vi "Draw Angle Line.vi"(9 "BG Image Property In":T1={"Radius"=[], "Plot Area Bounds"={"Left"=0, "Top"=0, "Right"=0, "Bottom"=0}, "Center position"={"X"=0, "Y"=0}, "Flip?"=FALSE, "Major Gird Color"=10066176, "Minor Gird Color"=5000192}, 11 "Picture In":picture) -> (1 "BG Image Property Out":T1={"Radius"=[], "Plot Area Bounds"={"Left"=0, "Top"=0, "Right"=0, "Bottom"=0}, "Center position"={"X"=0, "Y"=0}, "Flip?"=FALSE, "Major Gird Color"=10066176, "Minor Gird Color"=5000192}, 3 "Picture Out":picture)   [LabVIEW 2020, in "2D Compass.lvclass"]
uses:
  <vilib>/Math Plots/2D Math Plots/2D Compass/2D Compass/2D Compass.lvclass
  <vilib>/Math Plots/2D Math Plots/2D Compass/2D Compass/Typedef/BG Image Property.ctl
  <vilib>/Utility/miscctls.llb/LVRectTypeDef.ctl
panel:
  in  "Default Angle Array":cluster{"Angle":dbl, "Min Radius":i16}[](array[cluster])=[{"Angle"=0.0, "Min Radius"=0}, {"Angle"=15.0, "Min Radius"=25}, {"Angle"=30.0, "Min Radius"=25}, {"Angle"=45.0, "Min Radius"=10}, {"Angle"=60.0, "Min Radius"=25}, {"Angle"=75.0, "Min Radius"=25}]
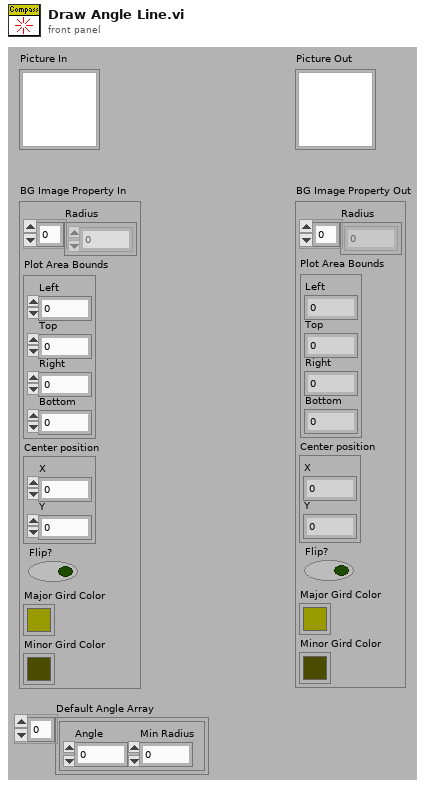
[diagram p1: front panel]
types:
  T1 = typedef "2D Compass.lvclass/BG Image Property.ctl" = cluster{"Radius":i16[], "Plot Area Bounds":T2, "Center position":cluster{"X":i16, "Y":i16}, "Flip?":bool, "Major Gird Color":u32, "Minor Gird Color":u32}
  T2 = typedef "LVRectTypeDef.ctl" = cluster{"Left":i16, "Top":i16, "Right":i16, "Bottom":i16}
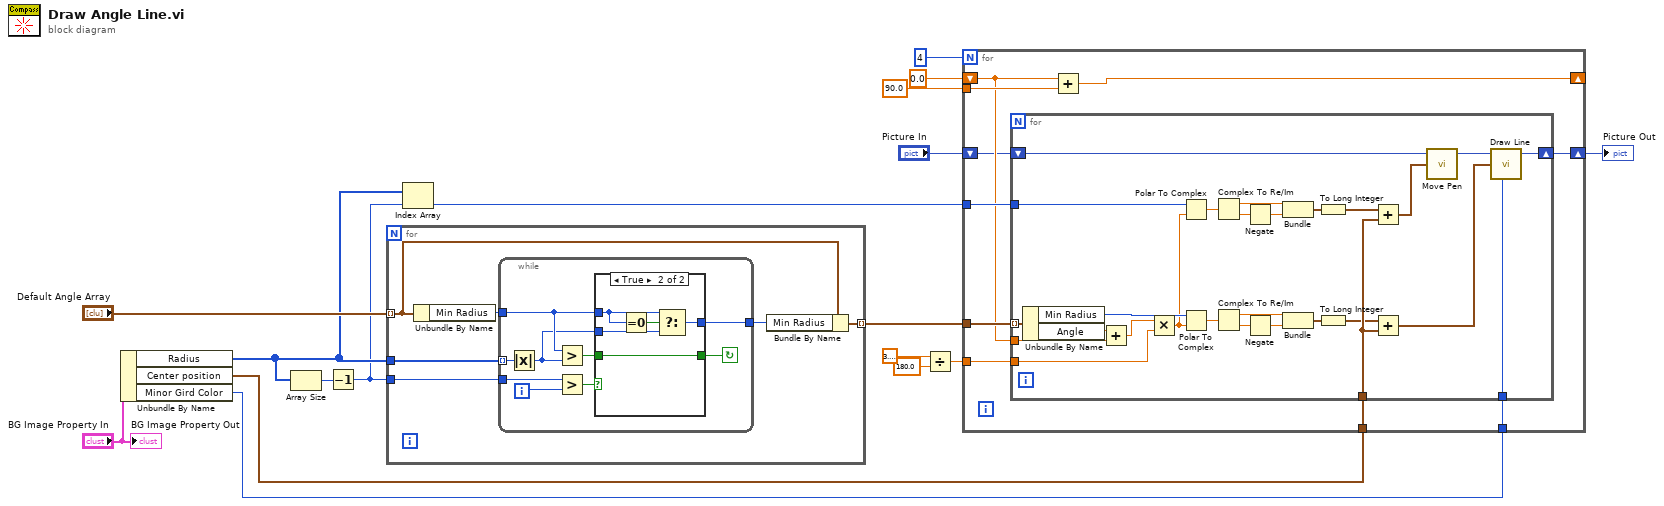
[diagram p0: block diagram]
diagram:
  n1 = Unbundle By Name("BG Image Property In") -> ("Radius"=w9:i16[], "Center position"=w3:cluster{"X":i16, "Y":i16}, "Minor Gird Color"=w4:u32)
  n2 = Array Size(array=w9) -> (size(s)=w16:i32)
  n3 = Decrement(x=w16) -> (x-1=w8:i32)
  n4 = for {
    tunnel: w9 -> [w21]
    tunnel: "Default Angle Array" -> [w23] mode=indexing
    tunnel: w8 -> [w22]
    tunnel: [w18] -> w10 mode=indexing
    n5 = Unbundle By Name(w23) -> ("Min Radius"=w20:i16)
    n6 = while {
      tunnel: [w27] -> w19
      tunnel: w20 -> [w26]
      tunnel: w22 -> [w31]
      tunnel: w21 -> [w24] mode=indexing
      i -> [w32]
      stop <- w29 continue-if-true
      n7 = Absolute Value(x=w24) -> (abs(x)=w25:i16)
      n8 = Greater?(x=w26, y=w25) -> (0:w28:bool)
      n9 = Greater?(x=w31, y=w32) -> (0:w30:bool)
      n10 = case shown="True" w30 {
        selector: w30 -> [w34 _]
        tunnel: [w34 w39] -> w29
        tunnel: w25 -> [w33 w35]
        tunnel: w28 -> [_ w39]
        tunnel: [w33 w36] -> w27
        tunnel: w26 -> [_ w37]
        frame False {
          # "last element"
        }
        frame True {
          n11 = Equal To 0?(x=w37) -> (x = 0?=w38:bool)
          n12 = Select(t=w37, s=w38, f=w35) -> (s? t:f=w36:i16)
        }
      }
    }
    n13 = Bundle By Name(cluster=w23, "Min Radius"=w19) -> (w18:cluster{"Angle":dbl, "Min Radius":i16})
  }
  n14 = Index Array(array=w9, index=w8) -> (element=w7:i16)
  n15 = Divide(x=3.141592653589793, y=180.0) -> (x/y=w14:dbl)
  n16 = for {
    N: 4 -> [_]
    shift-left: "Picture In" -> [w41]
    shift-right: [w40] -> w1
    tunnel: 90.0 -> [w43]
    tunnel: w4 -> [w44]
    tunnel: w3 -> [w45]
    tunnel: w10 -> [w46]
    tunnel: w7 -> [w47]
    tunnel: w14 -> [w48]
    shift-left: 0.0 -> [w42]
    shift-right: [w49] -> _
    n17 = for {
      tunnel: w46 -> [w76] mode=indexing
      shift-right: [w74] -> w40
      shift-left: w41 -> [w75]
      tunnel: w45 -> [w73]
      tunnel: w44 -> [w72]
      tunnel: w48 -> [w71]
      tunnel: w47 -> [w69]
      tunnel: w42 -> [w68]
      n18 = Unbundle By Name(w76) -> ("Min Radius"=w70:i16, "Angle"=w50:dbl)
      n19 = Add(x=w50, y=w68) -> (x+y=w67:dbl)
      n20 = Multiply(x=w67, y=w71) -> (x*y=w59:dbl)
      n21 = Polar To Complex(1:w59, 2:w69) -> (0:w58:cdb)
      n22 = Polar To Complex(1:w59, 2:w70) -> (0:w55:cdb)
      n23 = Complex To Re/Im(x + iy=w58) -> (x=w60:dbl, y=w61:dbl)
      n24 = Complex To Re/Im(x + iy=w55) -> (x=w56:dbl, y=w57:dbl)
      n25 = Negate(x=w61) -> (-x=w51:dbl)
      n26 = Negate(x=w57) -> (-x=w52:dbl)
      n27 = Bundle(w60, w51) -> (w53:cluster{dbl, dbl})  [unwired: 1 out]
      n28 = Bundle(w56, w52) -> (w54:cluster{dbl, dbl})  [unwired: 1 out]
      n29 = To Long Integer(number=w53) -> (32bit integer=w63:cluster{i32, i32})
      n30 = To Long Integer(number=w54) -> (32bit integer=w62:cluster{i32, i32})
      n31 = Add(x=w63, y=w73) -> (x+y=w65:cluster{i32, i32})
      n32 = Add(x=w62, y=w73) -> (x+y=w66:cluster{i32, i32})
      n33 = call <vilib>:"Move Pen.vi"("new position"=w65, "picture"=w75) -> ("new picture"=w64:picture)  [unwired: 1 in, 2 out]
      n34 = call <vilib>:"Draw Line.vi"("picture"=w64, "end point"=w66, "color(black)"=w72) -> ("new picture"=w74:picture)  [unwired: 2 in, 4 out]
    }
    n35 = Add(x=w42, y=w43) -> (x+y=w49:dbl)
  }
  "Picture Out" <- w1
  "BG Image Property Out" <- "BG Image Property In"
